vi "setAandPinvA.vi"(8 "error in (no error)":errorcluster, 9 "Truncation Threshold":dbl=0.0001, 10 "Field Idx":i32[](array[numeric]), 11 "OptStateEsti in":refnum<class "OptStateEsti.lvclass">) -> (0 "error out":errorcluster, 3 "OptStateEsti out":refnum<class "OptStateEsti.lvclass">)   [LabVIEW 2016, in "OptStateEsti.lvclass"]
doc: "Set the sensitivity matrix A and the related pseudo-inverse A^(-1)."
uses:
  OptStateEsti.lvclass
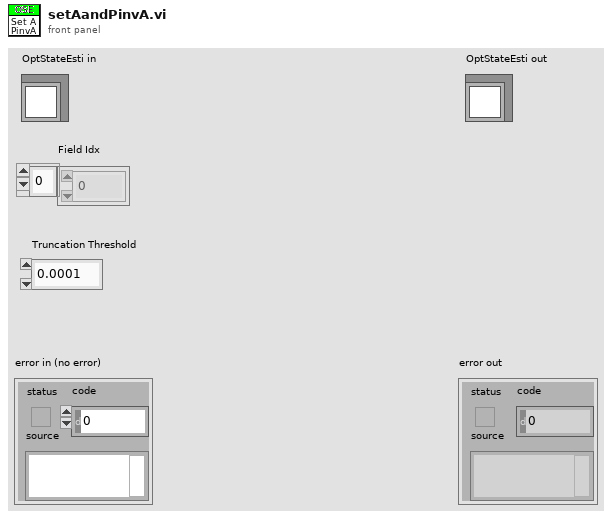
[diagram p1: front panel]
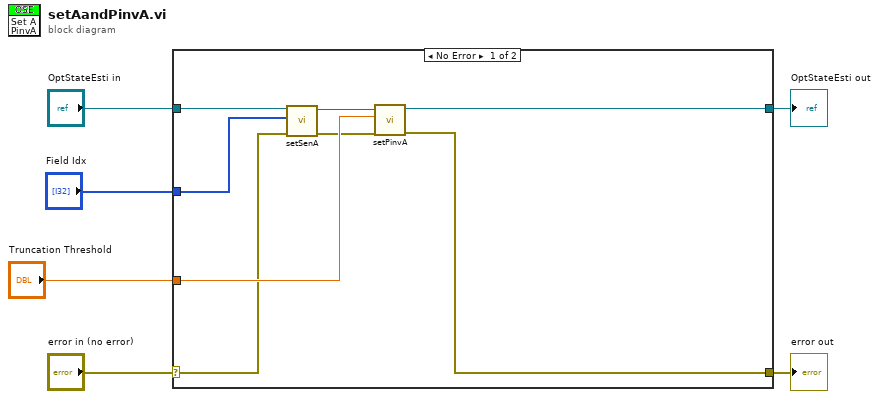
[diagram p0: block diagram]
diagram:
  n1 = case shown="No Error" "error in (no error)" {
    selector: "error in (no error)" -> [w9 w16]
    tunnel: [w7 w16] -> w5
    tunnel: [w11 w15] -> w3
    tunnel: "OptStateEsti in" -> [w14 w15]
    tunnel: "Field Idx" -> [w13 _]
    tunnel: "Truncation Threshold" -> [w10 _]
    frame No Error {
      n2 = call "setSenA.vi"("error in (no error)"=w9, "Field Idx"=w13, "OptStateEsti in"=w14) -> ("error out"=w8:errorcluster, "OptStateEsti out"=w12:refnum<class "OptStateEsti.lvclass">)  [unwired: 7 in]
      n3 = call "setPinvA.vi"("error in (no error)"=w8, "Truncation Threshold"=w10, "OptStateEsti in"=w12) -> ("error out"=w7:errorcluster, "OptStateEsti out"=w11:refnum<class "OptStateEsti.lvclass">)  [unwired: 7 in]
    }
    frame Error {
    }
  }
  "error out" <- w5
  "OptStateEsti out" <- w3
